vi "Get Random Salt.vi"(8 "error in (no error)":errorcluster, 11 "# of bytes (32)":i32=32) -> (0 "error out":errorcluster, 2 "random bytes":u8[](array[numeric]) format="%02x", 3 "hex salt":string)   [LabVIEW 2013]
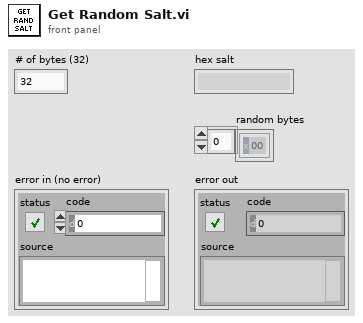
[diagram p1: front panel]
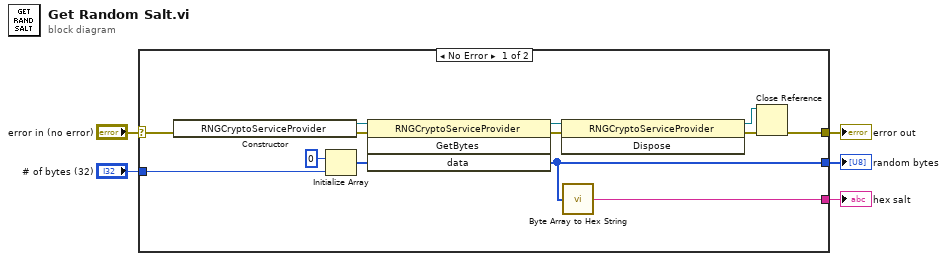
[diagram p0: block diagram]
diagram:
  n1 = case shown="No Error" "error in (no error)" {
    selector: "error in (no error)" -> [w7 w19]
    tunnel: "# of bytes (32)" -> [w17 _]
    tunnel: [w16 _] -> w4
    tunnel: [w8 _] -> w3
    tunnel: [w6 w19] -> w1
    frame No Error {
      n2 = constructor class="RNGCryptoServiceProvider"(error in=w7) -> (reference out=w15:refnum<k24>, error out=w14:errorcluster)  [unwired: 2 in, 1 out]
      n3 = Initialize Array(u8 0, w17) -> (w9:u8[])
      n4 = invoke class="RNGCryptoServiceProvider" method="GetBytes"(reference=w15, error in=w14, "data"=w9) -> (reference out=w13:refnum<k24>, error out=w12:errorcluster, "data"=w8:u8[])  [unwired: 1 in, 1 out]
      n5 = invoke class="RNGCryptoServiceProvider" method="Dispose"(reference=w13, error in=w12) -> (reference out=w10:refnum<k24>, error out=w11:errorcluster)  [unwired: 1 in, 1 out]
      n6 = call "Byte Array to Hex String.vi"("bytes array"=w8) -> ("hex string (normal display)"=w16:string)
      n7 = Close Reference(reference=w10, error in (no error)=w11) -> (error out=w6:errorcluster)
    }
    frame Error {
    }
  }
  "hex salt" <- w4
  "random bytes" <- w3
  "error out" <- w1
